vi "Identify Top Source Directory.vi"(8 "error in (no error)":errorcluster, 10 "Build Directory":path, 11 "Library Path":path) -> (0 "error out":errorcluster, 3 "Library Top-Level Path":string)   [LabVIEW 2019]
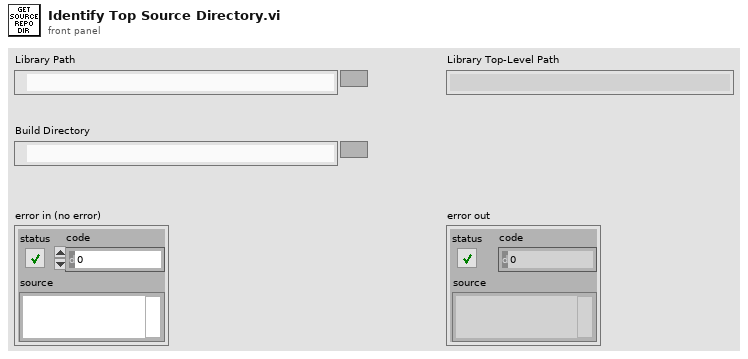
[diagram p1: front panel]
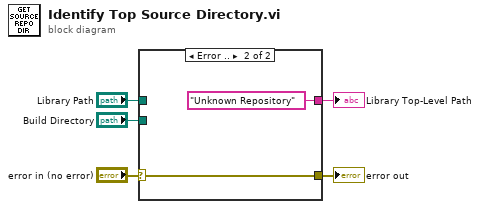
[diagram p0: block diagram]
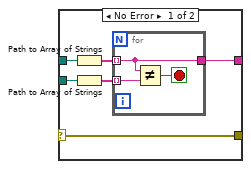
[diagram p2: hidden frame]
diagram:
  n1 = case shown="Error .." "error in (no error)" {
    selector: "error in (no error)" -> [w11 w16]
    tunnel: [w11 w16] -> w4
    tunnel: "Library Path" -> [w10 _]
    tunnel: "Build Directory" -> [w9 _]
    tunnel: [w6 "Unknown Repository"] -> w1
    frame No Error {
      n2 = Path to Array of Strings(0:w10) -> (2:w8:string[])  [unwired: 1 out]
      n3 = Path to Array of Strings(0:w9) -> (2:w7:string[])  [unwired: 1 out]
      n4 = for {
        tunnel: w8 -> [w12] mode=indexing
        tunnel: w7 -> [w14] mode=indexing
        tunnel: [w12] -> w6
        stop <- w13 stop-if-true
        n5 = Not Equal?(x=w12, y=w14) -> (x != y?=w13:bool)
      }
    }
    frame Error {
    }
  }
  "Library Top-Level Path" <- w1
  "error out" <- w4
